vi "Arduino_Upload.vi"(8 "error in (no error)":errorcluster, 10 "serial":string, 11 "Arduino In":T1={"Java"=path "/Applications/Arduino.app/Contents/Java", "Packages"=path "/Users/crogers/Library/Arduino15/packages", "folder"=path "/Users/crogers/Documents/LabVIEW Data", "serial"="/dev/cu.usbmodem14301", "Console"=""}) -> (0 "error out":errorcluster, 3 "Arduino Out":T1={"Java"=path "/Applications/Arduino.app/Contents/Java", "Packages"=path "/Users/crogers/Library/Arduino15/packages", "folder"=path "/Users/crogers/Documents/LabVIEW Data", "serial"="/dev/cu.usbmodem14301", "Console"=""})   [LabVIEW 2024]
uses:
  Arduino.ctl
panel:
  out "resulting string":string
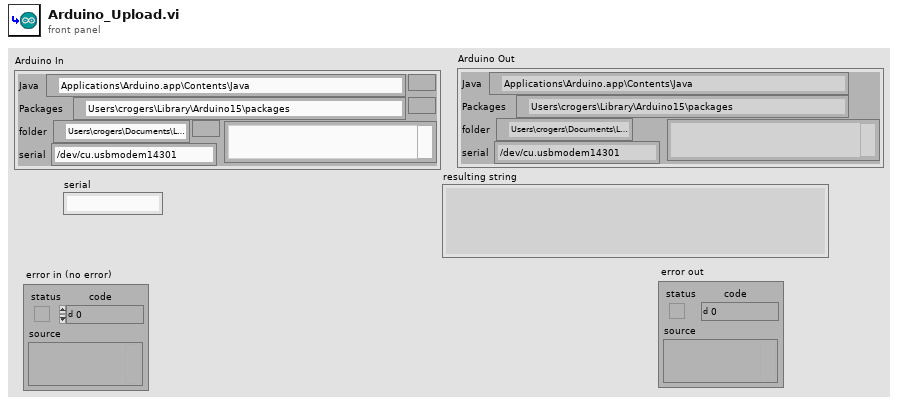
[diagram p1: front panel]
types:
  T1 = typedef "Arduino.ctl" = cluster{"Java":path, "Packages":path, "folder":path, "serial":string, "Console":string}
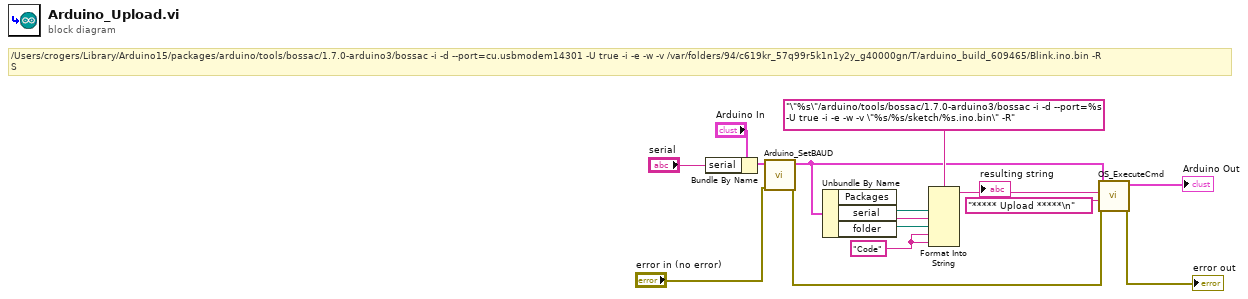
[diagram p0: block diagram]
diagram:
  w2 = "Code" ("Name")
  # "/Users/crogers/Library/Arduino15/packages/arduino/tools/bossac/1.7.0-arduino3/bossac -i -d --port=cu.usbmodem14301 -U true -i -e -w -v /var/folders/94/c619kr_57q99r5k1n1y2y_g40000gn/T/arduino_build_609465/Blink.ino.bin -R \nS"
  n1 = Bundle By Name(cluster="Arduino In", "serial"="serial") -> (w3:T1)
  n2 = call "Arduino_SetBAUD.vi"("error in (no error)"="error in (no error)", "Arduino In"=w3) -> ("error out"=w13:errorcluster, "Arduino Out"=w6:T1)  [unwired: 8 in]
  n3 = Unbundle By Name(w6) -> ("Packages"=w9:path, "serial"=w8:string, "folder"=w7:path)
  n4 = Format Into String(format string="\"%s\"/arduino/tools/bossac/1.7.0-arduino3/bossac -i -d --port=%s -U true -i -e -w -v \"%s/%s/sketch/%s.ino.bin\" -R" ("name or relative path"), w9, w8, w7, w2, w2) -> (resulting string=w11:string)  [unwired: 2 in, 1 out]
  "resulting string" <- w11
  n5 = call "OS_ExecuteCmd.vi"("error in (no error)"=w13, "Comment"="***** Upload *****\n" ("string"), "Command"=w11, "Arduino In"=w6) -> ("error out"=→"error out":errorcluster, "Arduino out"=→"Arduino Out":T1)  [unwired: 6 in]
